vi "Write Output Power.vi"(8 "error in":errorcluster, 10 "Power (uW)":dbl, 11 "LTB-1 in":refnum<class "LTB-1.lvclass">) -> (0 "error out":errorcluster, 3 "LTB-1 out":refnum<class "LTB-1.lvclass">)   [LabVIEW 2018, in "LTB-1.lvlib" / "LTB-1.lvclass"]
doc: "This is a dynamically dispatched VI. The child class will set the output power level in microWatts measured by the variable optical attenuator. VOA Power meter reports in dB - use appropriate equations to convert from dB to uW.\n\nAuthor: Ron Dexter\nCompany: Luminar\nModified: 5/20/2018"
uses:
  LTB-1.lvclass
  C:/AME Test Engineering/LabVIEW/PPLs/EXFO/Parent/EXFO.lvlibp/EXFO.lvclass
  LTB-1.lvclass/LTB-1.ctl
  PPLs/EXFO/Parent/EXFO.lvlibp/Methods/Read Resource.vi
  3150 Driver/3150.lvlib
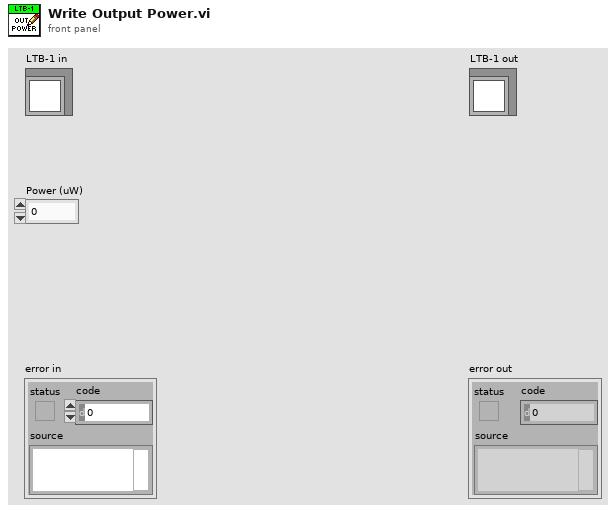
[diagram p1: front panel]
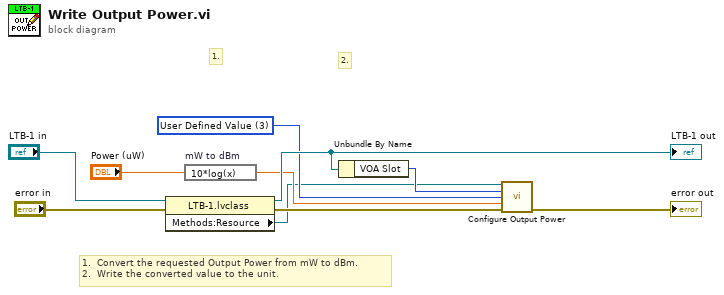
[diagram p0: block diagram]
diagram:
  w3 = 3 items=["MINimum", "MAXimum", "DEFault", "User Defined Value"] ("Output Power (0:MINimum)")
  # "1.  Convert the requested Output Power from mW to dBm.\n2.  Write the converted value to the unit."
  # "2."
  # "1."
  n1 = property class="LTB-1.lvclass"(reference="LTB-1 in", error in="error in") -> (reference out=w7:refnum<class "LTB-1.lvclass">, error out=w6:errorcluster, "Methods:Resource"=w1:refnum<visa-resource-name>)
  "LTB-1 out" <- w7
  n2 = expression code="10*log(x)" "mW to dBm"("Power (uW)") -> (w4:dbl)
  n3 = Unbundle By Name(w7) -> ("VOA Slot"=w2:i16)
  n4 = call "Configure Output Power.vi"("VISA resource name"=w1, "Platform Slot Number (10)"=w2, "Output Power (0:MINimum)"=w3, "User Defined Output Power Value (-15.000)"=w4, "error in (no error)"=w6) -> ("error out"=→"error out":errorcluster)  [unwired: 9 in, 1 out]
